vi "get_port.vi"(8 "error in (no error)":errorcluster, 11 "DL090602SutterMP285Stage in":refnum<class "StageDL090602SutterMP285.lvclass">) -> (0 "error out":errorcluster, 2 "serial port":refnum<visa-resource-name>, 3 "DL090602SutterMP285Stage out":refnum<class "StageDL090602SutterMP285.lvclass">)   [LabVIEW 2010, in "StageDL090602SutterMP285.lvclass"]
uses:
  StageDL090602SutterMP285.lvclass
  StageDL090602SutterMP285.lvclass/StageDL090602SutterMP285.ctl
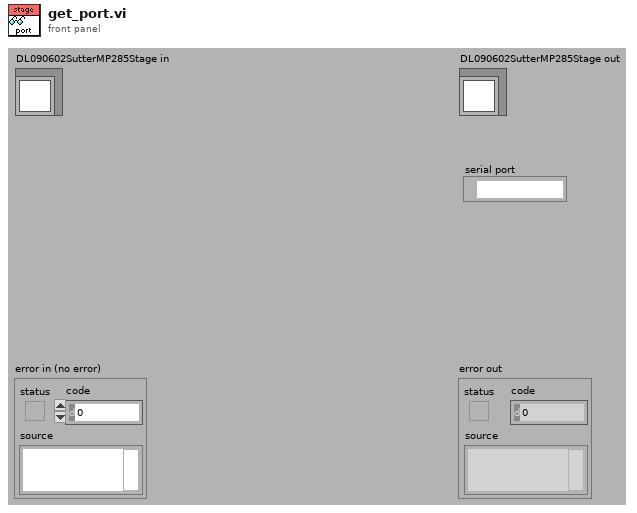
[diagram p1: front panel]
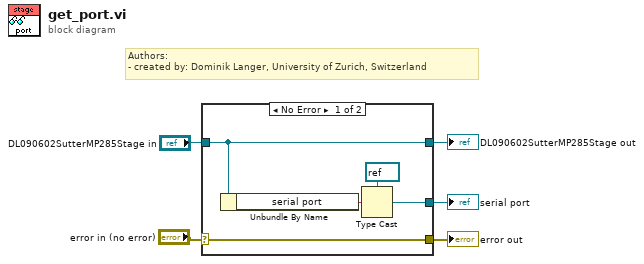
[diagram p0: block diagram]
diagram:
  # "Authors: \n- created by: Dominik Langer, University of Zurich, Switzerland"
  n1 = case shown="No Error" "error in (no error)" {
    selector: "error in (no error)" -> [w10 w12]
    tunnel: [w10 w12] -> w4
    tunnel: [w9 w11] -> w2
    tunnel: "DL090602SutterMP285Stage in" -> [w9 w11]
    tunnel: [w7 _] -> w1
    frame No Error {
      n2 = Unbundle By Name(w9) -> ("serial port"=w6:string)
      n3 = Type Cast(type=refnum<visa-resource-name> refnum ("VISA resource name"), x=w6) -> (*(type *) &x=w7:refnum<visa-resource-name>)
    }
    frame Error {
    }
  }
  "error out" <- w4
  "DL090602SutterMP285Stage out" <- w2
  "serial port" <- w1
